vi "test_DL950_fgv-simple.vi"() -> ()   [LabVIEW 2019]
uses:
  _ctrl/DL950_config.ctl
  _ctrl/fgv_DL950.ctl
  _ctrl/rw.ctl
panel:
  in  "config":T1={"Timeout"=10000, "Time Div"=12, "Acq Mode"=0, "Record Len"=0, "Record Num"=0, "Start Point"=0, "End Poin"=1000, "Visa"="", "Config Voltage"=[], "Trigger on"=FALSE, "Trigger Level"=0.0, "Reset"=FALSE, "Config Temp"=[], "Trigger Mode"=1, "Trigger Position"=50.0, "Trigger Slope"=0, "Trigger Source "=1, "Start Point (-5.00)"=-5.0, "End Point (5.00)"=5.0} {"End Point (5.00)" format="%.2g"; "Start Point (-5.00)" format="%.2f"; "Trigger Source" items=["", "CH1", "CH2", "CH3", "CH4", "CH5", "CH6", "CH7", "CH8", "CH9", "CH10", "CH11", "CH12", "CH13", "CH14", "CH15", "CH16", "RMATH1", "RMATH2", "RMATH3", "RMATH4", "RMATH5", "RMATH6", "RMATH7", "RMATH8", "RMATH9", "RMATH10", "RMATH11", "RMATH12", "RMATH13", "RMATH14", "RMATH15", "RMATH16"]; "Trigger Slope" items=["Rising", "Falling", "Both"]; "Trigger Position" format="%.1f"; "Trigger Mode" items=["Normal", "Auto", "Auto Level", "Single", "Single(N)", "On Start", "No Set"]; "Config Temp"."Type" items=["K", "E", "J", "T", "L", "U", "N", "R", "S", "B", "W", "Au7fe"]; "Config Temp"."Channel" items=["", "CH1", "CH2", "CH3", "CH4", "CH5", "CH6", "CH7", "CH8", "CH9", "CH10", "CH11", "CH12", "CH13", "CH14", "CH15", "CH16"]; "Trigger Level" format="%.3p"; "Config Voltage"."items" items=["Peak to Peak", "Amplitude", "Max", "Min", "High", "Low", "Average", "Middle", "Rms", "Standard Deviation", "+Overshoot", "-Overshoot", "Rise", "Fall", "Frequency", "Period", "+Width", "-Width", "Duty Cycle", "Pulse Count", "Burst1 Width", "Burst2 Width", "Average Frequency", "Average Period", "Int1TY", "Int2TY"]; "Config Voltage"."Probe" items=["1:1", "2:1", "5:1", "10:1", "20:1", "50:1", "100:1", "200:1", "500:1", "1000:1", "2000:1", "5000:1", "10k:1", "20k:1", "50k:1", "0.1A:1V", "0.2A:1V", "0.5A:1V", "1A:1V", "2A:1V", "5A:1V", "10A:1V", "20A:1V", "50A:1V", "100A:1V", "200A:1V", "250A:1V", "400A:1V", "500A:1V", "1kA:1V", "2kA:1V", "5kA:1V", "10kA:1V", "20kA:1V", "50kA:1V", "NoSet"]; "Config Voltage"."Ch" items=["None", "CH1", "CH2", "CH3", "CH4", "CH5", "CH6", "CH7", "CH8", "CH9", "CH10", "CH11", "CH12", "CH13", "CH14", "CH15", "CH16", "MATH1", "MATH2", "MATH3", "MATH4", "MATH5", "MATH6", "MATH7", "MATH8", "EVENT"]; "Config Voltage"."Coupling" items=["AC", "DC", "Ground", "AC-RMS", "DC-RMS"]; "Config Voltage"."V Div" items=["0.1m", "0.2m", "0.5m", "1m", "2m", "5m", "10m", "20m", "50m", "100m", "200m", "500m", "1", "2", "4", "5", "8", "10", "20", "40", "50", "80", "100", "200", "400", "500", "800", "1k", "2k", "4k", "5k", "8k", "10k", "20k", "25k", "50k", "100k", "250k", "500k", "1000k"]; "Record Len" items=["10k", "25k", "50k", "100k", "250k", "500k", "1M", "2.5M", "5M", "10M", "25M", "50M", "100M", "250M", "500M", "1G", "2G", "4G", "5G", "10G", "20G", "50G"]; "Acq Mode" items=["Normal", "Average", "Envelope"]; "Time Div" items=["100ns", "200ns", "500ns", "1us", "2us", "5us", "10us", "20us", "50us", "100us", "200us", "500us", "1ms", "2ms", "5ms", "10ms", "20ms", "50ms", "100ms", "200ms", "500ms", "1s", "2s", "3s", "4s", "5s", "6s", "10s", "20s", "30s", "1min", "2min", "3min", "4min", "5min", "6min", "10min", "12min", "30min", "1hour", "2hour", "3hour", "4hour", "5hour", "6hour", "8hour", "10hour", "12hour", "1day", "2day", "3day", "4day", "5day"]}
  out "ch1 graph":cluster{"l":dbl, "dt":dbl, "Y":dbl[][]}(graph)
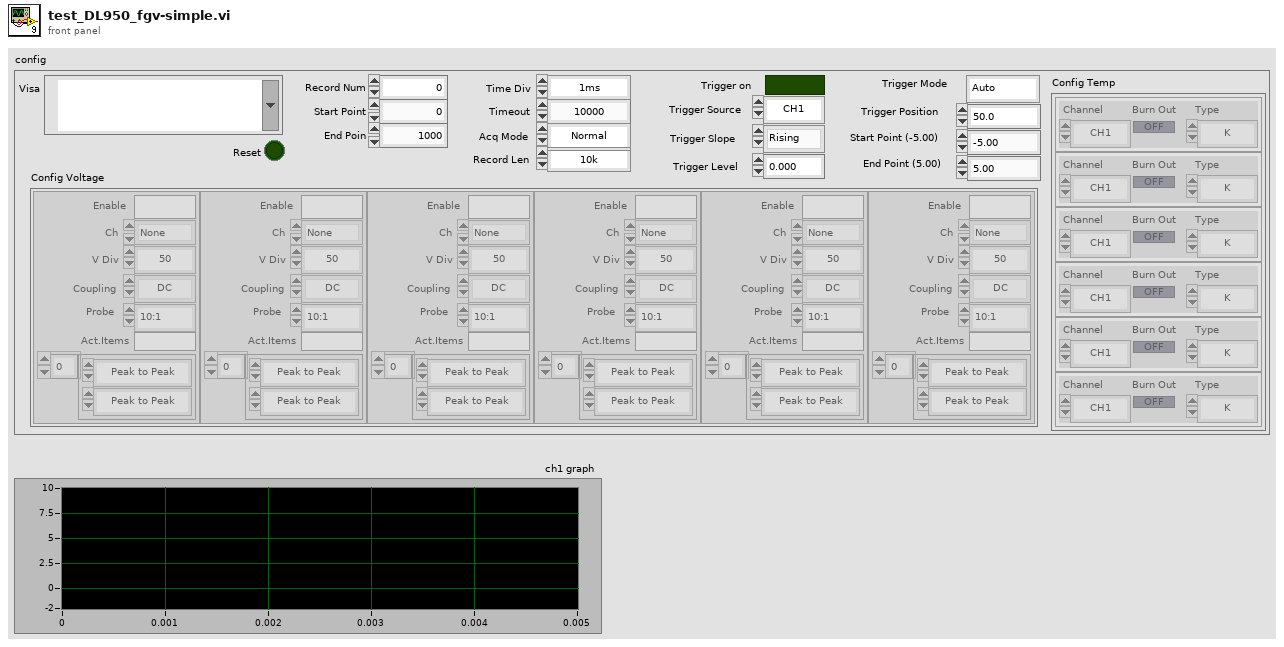
[diagram p1: front panel]
types:
  T1 = typedef "DL950_config.ctl" = cluster{"Timeout":u32, "Time Div":i32, "Acq Mode":i32, "Record Len":i32, "Record Num":i32, "Start Point":i64, "End Poin":i64, "Visa":refnum<visa-resource-name>, "Config Voltage":cluster{"Enable":bool, "Ch":u16, "V Div":i32, "Coupling":i32, "Probe":i32, "Act.Items":bool, "items":i32[]}[], "Trigger on":bool, "Trigger Level":dbl, "Reset":bool, "Config Temp":cluster{"Channel":u16, "Burn Out":bool, " Type ":i32}[], "Trigger Mode":i32, "Trigger Position":dbl, "Trigger Slope":i32, "Trigger Source ":i32, "Start Point (-5.00)":dbl, "End Point (5.00)":dbl}
  T2 = typedef "fgv_DL950.ctl" = enum16{"init", "config", "Set-NCh", "setapply", "trigger", "read", "time-div", "wave-aquis", "start", "query", "abort", "set_items", "reset_items", "read_items", "percent_rise", "trigger_single", "stop", "close"}
  T3 = typedef "rw.ctl" = enum16{"read", "write"}
  T4 = typedef "DL950_wfms.ctl" = cluster{"wfms":waveform(dbl)[], "Waveform_2":cluster{"t0":dbl, "dt":dbl, "Y":dbl[][]}}
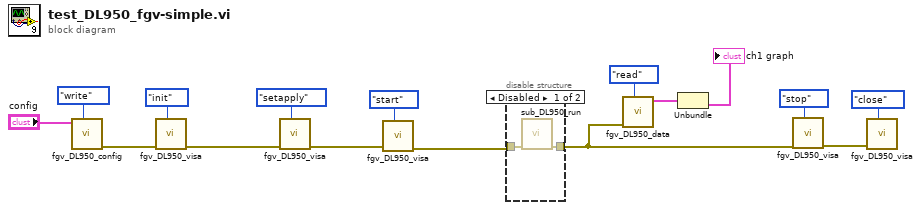
[diagram p0: block diagram]
diagram:
  n1 = call "fgv_DL950_config.vi"("cmd"=rw."write", "config"="config") -> ("error out"=w6:errorcluster)  [unwired: 8 in, 1 out]
  n2 = call "fgv_DL950_visa.vi"("cmd"=fgv_DL950."init", "error in"=w6) -> ("error out"=w4:errorcluster)  [unwired: 7 in, 2 out]
  n3 = call "fgv_DL950_visa.vi"("cmd"=fgv_DL950."setapply", "error in"=w4) -> ("error out"=w2:errorcluster)  [unwired: 7 in, 2 out]
  n4 = call "fgv_DL950_visa.vi"("cmd"=fgv_DL950."start", "error in"=w2) -> ("error out"=w1:errorcluster)  [unwired: 7 in, 2 out]
  n5 = disable-structure shown="Disabled" {
    disable-tunnel: w1 -> [w18 w19]
    disable-tunnel: [w17 w19] -> w5
    frame Disabled {
      n6 = call "sub_DL950_run.vi"("error in"=w18) -> ("error out"=w17:errorcluster)  [unwired: 10 in]
    }
    frame Enabled {
    }
  }
  n7 = call "fgv_DL950_data.vi"("cmd"=rw."read", "error in"=w5) -> ("DL950 wfm 2"=w10:T4)  [unwired: 8 in, 1 out]
  n8 = Unbundle(w10) -> ("Waveform_2"=→"ch1 graph":cluster{"t0":dbl, "dt":dbl, "Y":dbl[][]})  [unwired: 1 out]
  n9 = call "fgv_DL950_visa.vi"("cmd"=fgv_DL950."stop", "error in"=w5) -> ("error out"=w13:errorcluster)  [unwired: 7 in, 2 out]
  n10 = call "fgv_DL950_visa.vi"("cmd"=fgv_DL950."close", "error in"=w13) -> ()  [unwired: 7 in, 3 out]
